vi "统计合格率.vi"() -> ()   [LabVIEW 2010]
uses:
  全局量/试验配置信息.vi
  全局量/自动测试结果.vi
panel:
  in  "自测序号":i32
  in  "LAN合格路数":i32
  in  "RS485合格路数":i32
  in  "RS232合格路数":i32
  in  "CAN合格路数":i32
  in  "模拟量AD合格路数":i32
  in  "模拟量DSP合格路数":i32
  in  "数字量输出合格路数":i32
  in  "数字量输入合格路数":i32
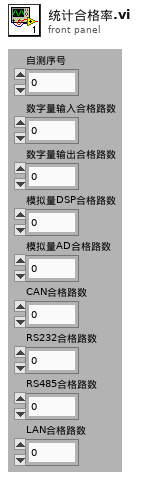
[diagram p1: front panel]
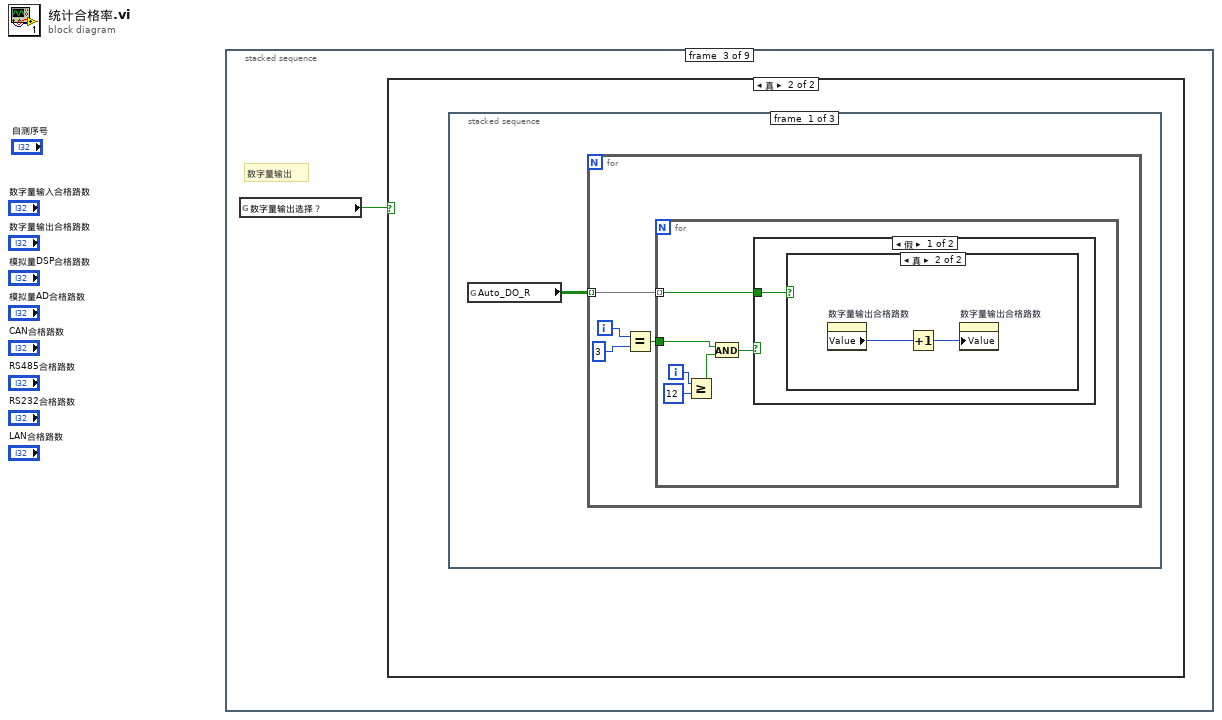
[diagram p0: block diagram]
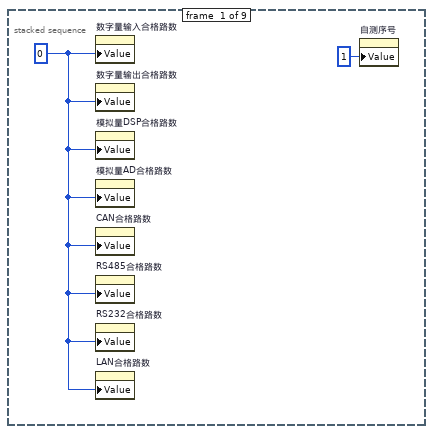
[diagram p2: hidden frame]
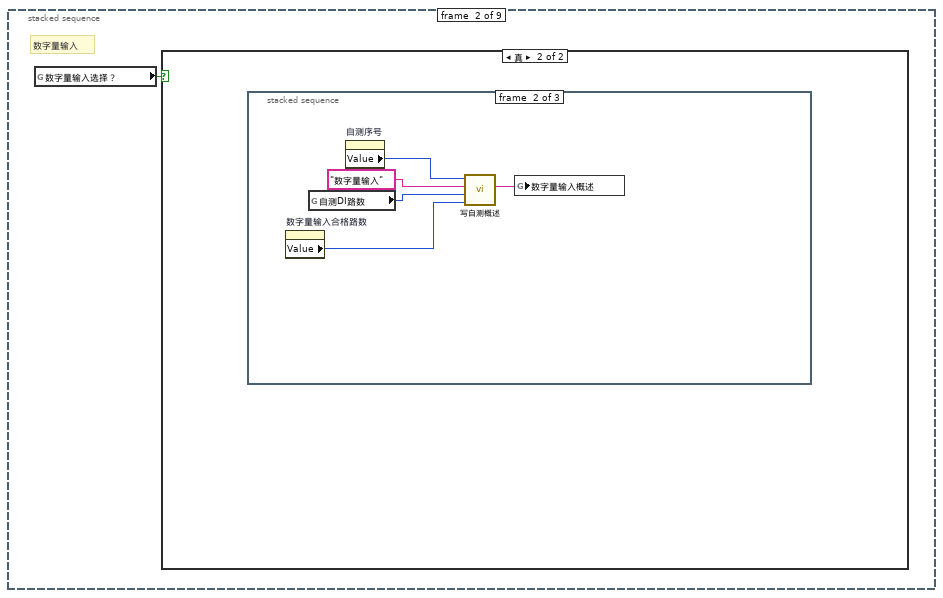
[diagram p3: hidden frame]
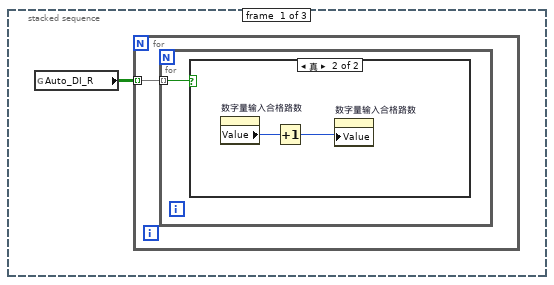
[diagram p5: hidden frame]
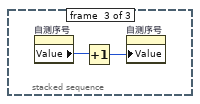
[diagram p7: hidden frame]
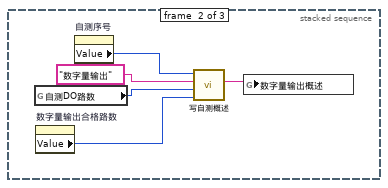
[diagram p11: hidden frame]
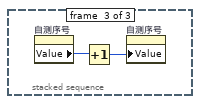
[diagram p12: hidden frame]
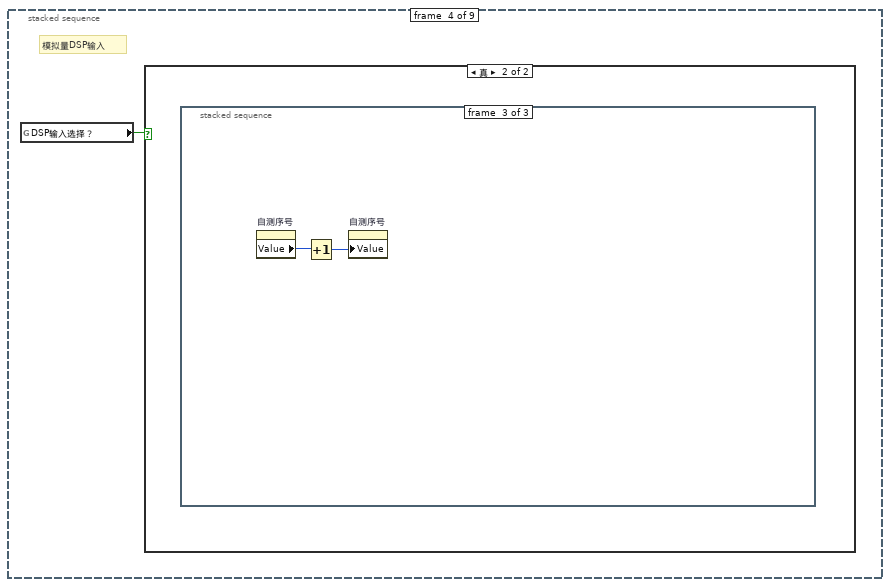
[diagram p13: hidden frame]
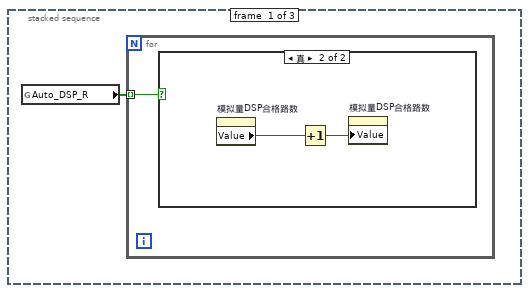
[diagram p15: hidden frame]
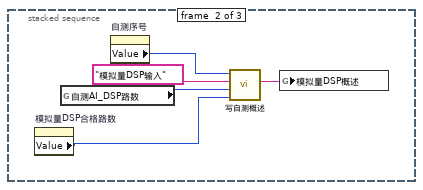
[diagram p17: hidden frame]
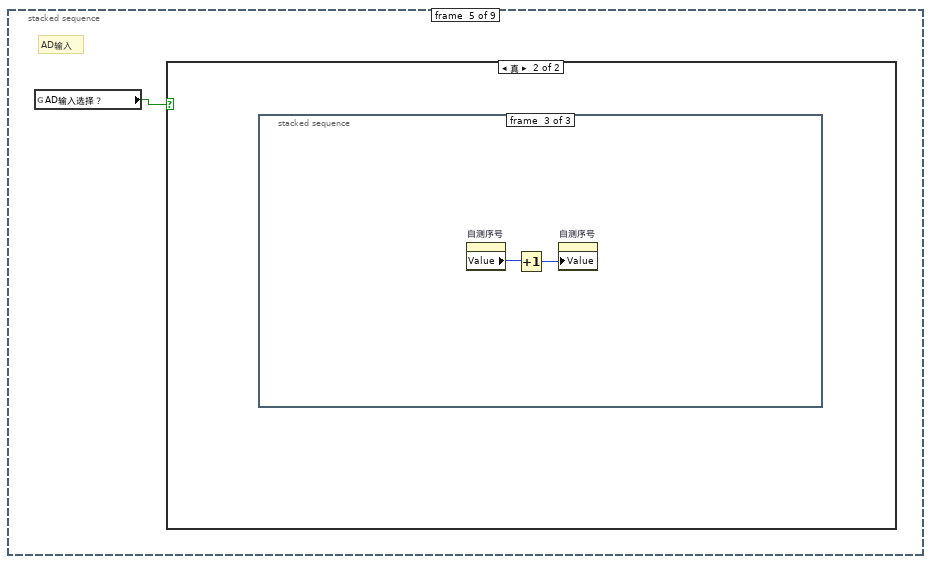
[diagram p18: hidden frame]
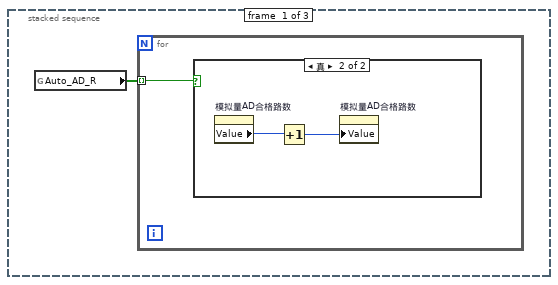
[diagram p20: hidden frame]
diagram:
  n1 = stacked-sequence {
    frame #0 {
      w2 = 0 ("数字量输入合格路数")
      n2 = property on="数字量输入合格路数" class="DigNum (严格)"("Value"=w2) -> ()  [unwired: 2 in, 2 out]
      n3 = property on="数字量输出合格路数" class="DigNum (严格)"("Value"=w2) -> ()  [unwired: 2 in, 2 out]
      n4 = property on="模拟量DSP合格路数" class="DigNum (严格)"("Value"=w2) -> ()  [unwired: 2 in, 2 out]
      n5 = property on="模拟量AD合格路数" class="DigNum (严格)"("Value"=w2) -> ()  [unwired: 2 in, 2 out]
      n6 = property on="CAN合格路数" class="DigNum (严格)"("Value"=w2) -> ()  [unwired: 2 in, 2 out]
      n7 = property on="RS485合格路数" class="DigNum (严格)"("Value"=w2) -> ()  [unwired: 2 in, 2 out]
      n8 = property on="RS232合格路数" class="DigNum (严格)"("Value"=w2) -> ()  [unwired: 2 in, 2 out]
      n9 = property on="LAN合格路数" class="DigNum (严格)"("Value"=w2) -> ()  [unwired: 2 in, 2 out]
      n10 = property on="自测序号" class="DigNum (严格)"("Value"=1 ("自测序号")) -> ()  [unwired: 2 in, 2 out]
    }
    frame #1 {
      # "数字量输入"
      n11 = global read "试验配置信息.vi" "数字量输入选择？"() -> (w3:bool)
      n12 = case shown="真" w3 {
        frame False {
        }
        frame True {
          n13 = stacked-sequence {
            frame #0 {
              n14 = global read "自动测试结果.vi" "Auto_DI_R"() -> (w4:bool[][])
              n15 = for {
                tunnel: w4 -> [w5] mode=indexing
                n16 = for {
                  tunnel: w5 -> [w6] mode=indexing
                  n17 = case shown="真" w6 {
                    frame False {
                    }
                    frame True {
                      n18 = property on="数字量输入合格路数" class="DigNum (严格)"() -> ("Value"=w7:i32)  [unwired: 2 in, 2 out]
                      n19 = Increment(x=w7) -> (x+1=w8:i32)
                      n20 = property on="数字量输入合格路数" class="DigNum (严格)"("Value"=w8) -> ()  [unwired: 2 in, 2 out]
                    }
                  }
                }
              }
            }
            frame #1 {
              n21 = property on="数字量输入合格路数" class="DigNum (严格)"() -> ("Value"=w10:i32)  [unwired: 2 in, 2 out]
              n22 = global read "试验配置信息.vi" "自测DI路数"() -> (w11:i32)
              n23 = property on="自测序号" class="DigNum (严格)"() -> ("Value"=w13:i32)  [unwired: 2 in, 2 out]
              n24 = call "写自测概述.vi"("合格路数"=w10, "共路数"=w11, "测试事项"="数字量输入", "自测序号"=w13) -> ("概述字符串"=w9:string)  [unwired: 7 in]
              n25 = global write "自动测试结果.vi" "数字量输入概述"(w9) -> ()
            }
            frame #2 {
              n26 = property on="自测序号" class="DigNum (严格)"() -> ("Value"=w14:i32)  [unwired: 2 in, 2 out]
              n27 = Increment(x=w14) -> (x+1=w15:i32)
              n28 = property on="自测序号" class="DigNum (严格)"("Value"=w15) -> ()  [unwired: 2 in, 2 out]
            }
          }
        }
      }
    }
    frame #2 {
      # "数字量输出"
      n29 = global read "试验配置信息.vi" "数字量输出选择？"() -> (w16:bool)
      n30 = case shown="真" w16 {
        frame False {
        }
        frame True {
          n31 = stacked-sequence {
            frame #0 {
              n32 = global read "自动测试结果.vi" "Auto_DO_R"() -> (w17:bool[][])
              n33 = for {
                tunnel: w17 -> [w21] mode=indexing
                i -> [w20]
                n34 = Equal?(x=w20, y=3) -> (x = y?=w18:bool)
                n35 = for {
                  tunnel: w21 -> [w27] mode=indexing
                  tunnel: w18 -> [w23]
                  i -> [w26]
                  n36 = Greater Or Equal?(x=w26, y=12) -> (x >= y?=w24:bool)
                  n37 = And(x=w23, y=w24) -> (x .and. y?=w22:bool)
                  n38 = case shown="假" w22 {
                    tunnel: w27 -> [w28 _]
                    frame False {
                      n39 = case shown="真" w28 {
                        frame False {
                        }
                        frame True {
                          n40 = property on="数字量输出合格路数" class="DigNum (严格)"() -> ("Value"=w29:i32)  [unwired: 2 in, 2 out]
                          n41 = Increment(x=w29) -> (x+1=w30:i32)
                          n42 = property on="数字量输出合格路数" class="DigNum (严格)"("Value"=w30) -> ()  [unwired: 2 in, 2 out]
                        }
                      }
                    }
                    frame True {
                    }
                  }
                }
              }
            }
            frame #1 {
              n43 = global read "试验配置信息.vi" "自测DO路数"() -> (w35:i32)
              n44 = property on="数字量输出合格路数" class="DigNum (严格)"() -> ("Value"=w32:i32)  [unwired: 2 in, 2 out]
              n45 = property on="自测序号" class="DigNum (严格)"() -> ("Value"=w33:i32)  [unwired: 2 in, 2 out]
              n46 = call "写自测概述.vi"("合格路数"=w32, "共路数"=w35, "测试事项"="数字量输出", "自测序号"=w33) -> ("概述字符串"=w31:string)  [unwired: 7 in]
              n47 = global write "自动测试结果.vi" "数字量输出概述"(w31) -> ()
            }
            frame #2 {
              n48 = property on="自测序号" class="DigNum (严格)"() -> ("Value"=w37:i32)  [unwired: 2 in, 2 out]
              n49 = Increment(x=w37) -> (x+1=w36:i32)
              n50 = property on="自测序号" class="DigNum (严格)"("Value"=w36) -> ()  [unwired: 2 in, 2 out]
            }
          }
        }
      }
    }
    frame #3 {
      # "模拟量DSP输入"
      n51 = global read "试验配置信息.vi" "DSP输入选择？"() -> (w38:bool)
      n52 = case shown="真" w38 {
        frame False {
        }
        frame True {
          n53 = stacked-sequence {
            frame #0 {
              n54 = global read "自动测试结果.vi" "Auto_DSP_R"() -> (w39:bool[])
              n55 = for {
                tunnel: w39 -> [w40] mode=indexing
                n56 = case shown="真" w40 {
                  frame False {
                  }
                  frame True {
                    n57 = property on="模拟量DSP合格路数" class="DigNum (严格)"() -> ("Value"=w41:i32)  [unwired: 2 in, 2 out]
                    n58 = Increment(x=w41) -> (x+1=w42:i32)
                    n59 = property on="模拟量DSP合格路数" class="DigNum (严格)"("Value"=w42) -> ()  [unwired: 2 in, 2 out]
                  }
                }
              }
            }
            frame #1 {
              n60 = property on="模拟量DSP合格路数" class="DigNum (严格)"() -> ("Value"=w43:i32)  [unwired: 2 in, 2 out]
              n61 = global read "试验配置信息.vi" "自测AI_DSP路数"() -> (w46:i32)
              n62 = property on="自测序号" class="DigNum (严格)"() -> ("Value"=w44:i32)  [unwired: 2 in, 2 out]
              n63 = call "写自测概述.vi"("合格路数"=w43, "共路数"=w46, "测试事项"="模拟量DSP输入", "自测序号"=w44) -> ("概述字符串"=w47:string)  [unwired: 7 in]
              n64 = global write "自动测试结果.vi" "模拟量DSP概述"(w47) -> ()
            }
            frame #2 {
              n65 = property on="自测序号" class="DigNum (严格)"() -> ("Value"=w48:i32)  [unwired: 2 in, 2 out]
              n66 = Increment(x=w48) -> (x+1=w49:i32)
              n67 = property on="自测序号" class="DigNum (严格)"("Value"=w49) -> ()  [unwired: 2 in, 2 out]
            }
          }
        }
      }
    }
    frame #4 {
      # "AD输入"
      n68 = global read "试验配置信息.vi" "AD输入选择？"() -> (w50:bool)
      n69 = case shown="真" w50 {
        frame False {
        }
        frame True {
          n70 = stacked-sequence {
            frame #0 {
              n71 = global read "自动测试结果.vi" "Auto_AD_R"() -> (w51:bool[])
              n72 = for {
                tunnel: w51 -> [w52] mode=indexing
                n73 = case shown="真" w52 {
                  frame False {
                  }
                  frame True {
                    n74 = property on="模拟量AD合格路数" class="DigNum (严格)"() -> ("Value"=w54:i32)  [unwired: 2 in, 2 out]
                    n75 = Increment(x=w54) -> (x+1=w53:i32)
                    n76 = property on="模拟量AD合格路数" class="DigNum (严格)"("Value"=w53) -> ()  [unwired: 2 in, 2 out]
                  }
                }
              }
            }
            frame #1 {
              n77 = global read "试验配置信息.vi" "自测AI_AD路数"() -> (w57:i32)
              n78 = property on="模拟量AD合格路数" class="DigNum (严格)"() -> ("Value"=w55:i32)  [unwired: 2 in, 2 out]
              n79 = property on="自测序号" class="DigNum (严格)"() -> ("Value"=w59:i32)  [unwired: 2 in, 2 out]
              n80 = call "写自测概述.vi"("合格路数"=w55, "共路数"=w57, "测试事项"="模拟量AD输入", "自测序号"=w59) -> ("概述字符串"=w56:string)  [unwired: 7 in]
              n81 = global write "自动测试结果.vi" "模拟量AD概述结果"(w56) -> ()
            }
            frame #2 {
              n82 = property on="自测序号" class="DigNum (严格)"() -> ("Value"=w60:i32)  [unwired: 2 in, 2 out]
              n83 = Increment(x=w60) -> (x+1=w61:i32)
              n84 = property on="自测序号" class="DigNum (严格)"("Value"=w61) -> ()  [unwired: 2 in, 2 out]
            }
          }
        }
      }
    }
    frame #5 {
      # "CAN总线测试"
      n85 = global read "试验配置信息.vi" "CAN选择？"() -> (w62:bool)
      n86 = case shown="真" w62 {
        frame False {
        }
        frame True {
          n87 = stacked-sequence {
            frame #0 {
              n88 = global read "自动测试结果.vi" "Auto_CAN_R"() -> (w63:bool[])
              n89 = for {
                tunnel: w63 -> [w64] mode=indexing
                n90 = case shown="真" w64 {
                  frame False {
                  }
                  frame True {
                    n91 = property on="CAN合格路数" class="DigNum (严格)"() -> ("Value"=w66:i32)  [unwired: 2 in, 2 out]
                    n92 = Increment(x=w66) -> (x+1=w65:i32)
                    n93 = property on="CAN合格路数" class="DigNum (严格)"("Value"=w65) -> ()  [unwired: 2 in, 2 out]
                  }
                }
              }
            }
            frame #1 {
              n94 = property on="CAN合格路数" class="DigNum (严格)"() -> ("Value"=w67:i32)  [unwired: 2 in, 2 out]
              n95 = global read "试验配置信息.vi" "自测CAN路数"() -> (w69:i32)
              n96 = property on="自测序号" class="DigNum (严格)"() -> ("Value"=w71:i32)  [unwired: 2 in, 2 out]
              n97 = call "写自测概述.vi"("合格路数"=w67, "共路数"=w69, "测试事项"="CAN通讯测试", "自测序号"=w71) -> ("概述字符串"=w68:string)  [unwired: 7 in]
              n98 = global write "自动测试结果.vi" "CAN测试概述"(w68) -> ()
            }
            frame #2 {
              n99 = property on="自测序号" class="DigNum (严格)"() -> ("Value"=w72:i32)  [unwired: 2 in, 2 out]
              n100 = Increment(x=w72) -> (x+1=w73:i32)
              n101 = property on="自测序号" class="DigNum (严格)"("Value"=w73) -> ()  [unwired: 2 in, 2 out]
            }
          }
        }
      }
    }
    frame #6 {
      # "RS232"
      n102 = global read "试验配置信息.vi" "RS232选择？"() -> (w74:bool)
      n103 = case shown="真" w74 {
        frame False {
        }
        frame True {
          n104 = stacked-sequence {
            frame #0 {
              n105 = global read "自动测试结果.vi" "Auto_RS232_R"() -> (w75:bool[])
              n106 = for {
                tunnel: w75 -> [w76] mode=indexing
                n107 = case shown="真" w76 {
                  frame False {
                  }
                  frame True {
                    n108 = property on="RS232合格路数" class="DigNum (严格)"() -> ("Value"=w78:i32)  [unwired: 2 in, 2 out]
                    n109 = Increment(x=w78) -> (x+1=w77:i32)
                    n110 = property on="RS232合格路数" class="DigNum (严格)"("Value"=w77) -> ()  [unwired: 2 in, 2 out]
                  }
                }
              }
            }
            frame #1 {
              n111 = global read "试验配置信息.vi" "自测RS232路数"() -> (w81:i32)
              n112 = property on="RS232合格路数" class="DigNum (严格)"() -> ("Value"=w79:i32)  [unwired: 2 in, 2 out]
              n113 = property on="自测序号" class="DigNum (严格)"() -> ("Value"=w83:i32)  [unwired: 2 in, 2 out]
              n114 = call "写自测概述.vi"("合格路数"=w79, "共路数"=w81, "测试事项"="串口RS232通讯", "自测序号"=w83) -> ("概述字符串"=w80:string)  [unwired: 7 in]
              n115 = global write "自动测试结果.vi" "串口RS232测试概述"(w80) -> ()
            }
            frame #2 {
              n116 = property on="自测序号" class="DigNum (严格)"() -> ("Value"=w84:i32)  [unwired: 2 in, 2 out]
              n117 = Increment(x=w84) -> (x+1=w85:i32)
              n118 = property on="自测序号" class="DigNum (严格)"("Value"=w85) -> ()  [unwired: 2 in, 2 out]
            }
          }
        }
      }
    }
    frame #7 {
      # "RS485"
      n119 = global read "试验配置信息.vi" "RS485选择？"() -> (w86:bool)
      n120 = case shown="真" w86 {
        frame False {
        }
        frame True {
          n121 = stacked-sequence {
            frame #0 {
              n122 = global read "自动测试结果.vi" "Auto_RS485_R"() -> (w87:bool[])
              n123 = for {
                tunnel: w87 -> [w88] mode=indexing
                n124 = case shown="真" w88 {
                  frame False {
                  }
                  frame True {
                    n125 = property on="RS485合格路数" class="DigNum (严格)"() -> ("Value"=w89:i32)  [unwired: 2 in, 2 out]
                    n126 = Increment(x=w89) -> (x+1=w90:i32)
                    n127 = property on="RS485合格路数" class="DigNum (严格)"("Value"=w90) -> ()  [unwired: 2 in, 2 out]
                  }
                }
              }
            }
            frame #1 {
              n128 = property on="RS485合格路数" class="DigNum (严格)"() -> ("Value"=w91:i32)  [unwired: 2 in, 2 out]
              n129 = global read "试验配置信息.vi" "自测485路数"() -> (w93:i32)
              n130 = property on="自测序号" class="DigNum (严格)"() -> ("Value"=w95:i32)  [unwired: 2 in, 2 out]
              n131 = call "写自测概述.vi"("合格路数"=w91, "共路数"=w93, "测试事项"="串口RS485通讯", "自测序号"=w95) -> ("概述字符串"=w92:string)  [unwired: 7 in]
              n132 = global write "自动测试结果.vi" "串口RS485测试概述"(w92) -> ()
            }
            frame #2 {
              n133 = property on="自测序号" class="DigNum (严格)"() -> ("Value"=w96:i32)  [unwired: 2 in, 2 out]
              n134 = Increment(x=w96) -> (x+1=w97:i32)
              n135 = property on="自测序号" class="DigNum (严格)"("Value"=w97) -> ()  [unwired: 2 in, 2 out]
            }
          }
        }
      }
    }
    frame #8 {
      # "LAN"
      n136 = global read "试验配置信息.vi" "LAN选择？"() -> (w98:bool)
      n137 = case shown="真" w98 {
        frame False {
        }
        frame True {
          n138 = stacked-sequence {
            frame #0 {
              n139 = global read "自动测试结果.vi" "Auto_LAN_R"() -> (w99:bool)
              n140 = case shown="真" w99 {
                frame False {
                }
                frame True {
                  n141 = property on="LAN合格路数" class="DigNum (严格)"() -> ("Value"=w101:i32)  [unwired: 2 in, 2 out]
                  n142 = Increment(x=w101) -> (x+1=w100:i32)
                  n143 = property on="LAN合格路数" class="DigNum (严格)"("Value"=w100) -> ()  [unwired: 2 in, 2 out]
                }
              }
            }
            frame #1 {
              n144 = global read "试验配置信息.vi" "自测LAN路数"() -> (w104:i32)
              n145 = property on="LAN合格路数" class="DigNum (严格)"() -> ("Value"=w102:i32)  [unwired: 2 in, 2 out]
              n146 = property on="自测序号" class="DigNum (严格)"() -> ("Value"=w106:i32)  [unwired: 2 in, 2 out]
              n147 = call "写自测概述.vi"("合格路数"=w102, "共路数"=w104, "测试事项"="以太网通讯测试", "自测序号"=w106) -> ("概述字符串"=w103:string)  [unwired: 7 in]
              n148 = global write "自动测试结果.vi" "以太网测试概述"(w103) -> ()
            }
            frame #2 {
              n149 = property on="自测序号" class="DigNum (严格)"() -> ("Value"=w107:i32)  [unwired: 2 in, 2 out]
              n150 = Increment(x=w107) -> (x+1=w108:i32)
              n151 = property on="自测序号" class="DigNum (严格)"("Value"=w108) -> ()  [unwired: 2 in, 2 out]
            }
          }
        }
      }
    }
  }
